vi "calc centroid predict and correct.vi"(0 "Queue in":refnum<queue>, 1 "Session Out":T2, 5 "# Images in Burst":i32, 11 "error in (no error)":errorcluster) -> (15 "error out":errorcluster)   [LabVIEW 2020]
uses:
  <vilib>/vision/Image Controls.llb/IMAQ Image.ctl
  <vilib>/userdefined/High Color/IMAQdx.ctl
  <vilib>/vision/driver/NI_Vision_Acquisition_Software.lvlib
panel:
  in  "Tab Control":enum32{"Page 1", "Page 2"}(tab)
  in  "Range":cluster{"Lower value":sgl, "Upper value":sgl}={"Lower value"=128.0, "Upper value"=255.0} caption="Threshold Range" {"Upper value" format="%.2f"; "Lower value" format="%.2f"}
  in  "Use threshold fraction":bool=TRUE
  out "Waveform Chart":T1(graph)
  out "Images Processed":u32
  out "# elements in queue":i32
  out "Current Buffer Number":u32
  out "processed in burst":u32
  in  "threshold fraction":sgl=0.8
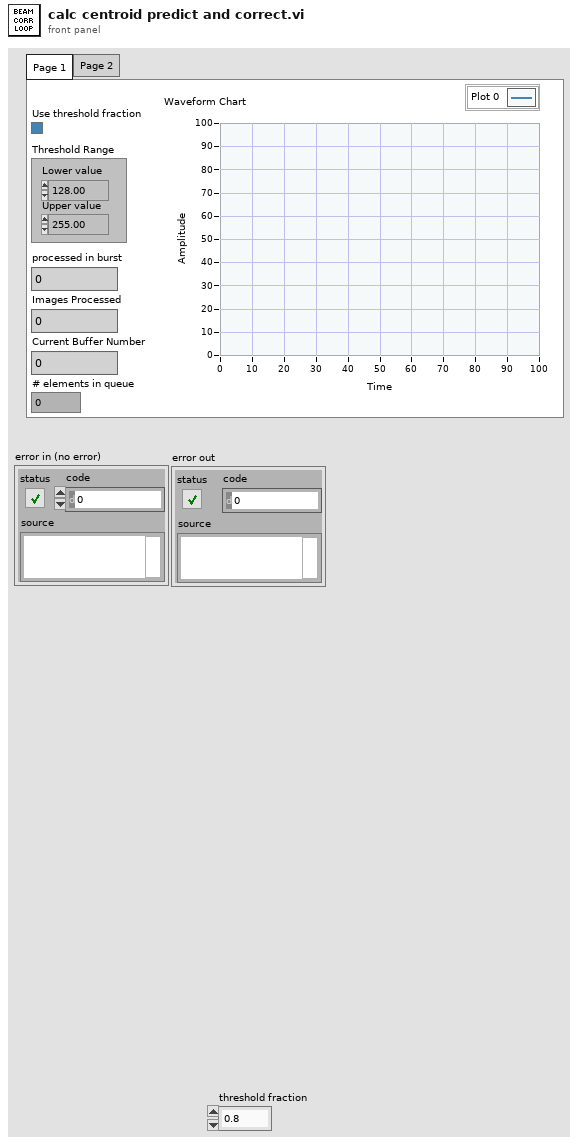
[diagram p1: front panel]
types:
  T1 = cluster{"X Centroid":sgl, "Y Centroid":sgl, "X Centroid":sgl, "Y Centroid":sgl}
  T2 = typedef "IMAQdx.ctl" = refnum<k21>
  T3 = typedef "IMAQ Image.ctl" = refnum<image>
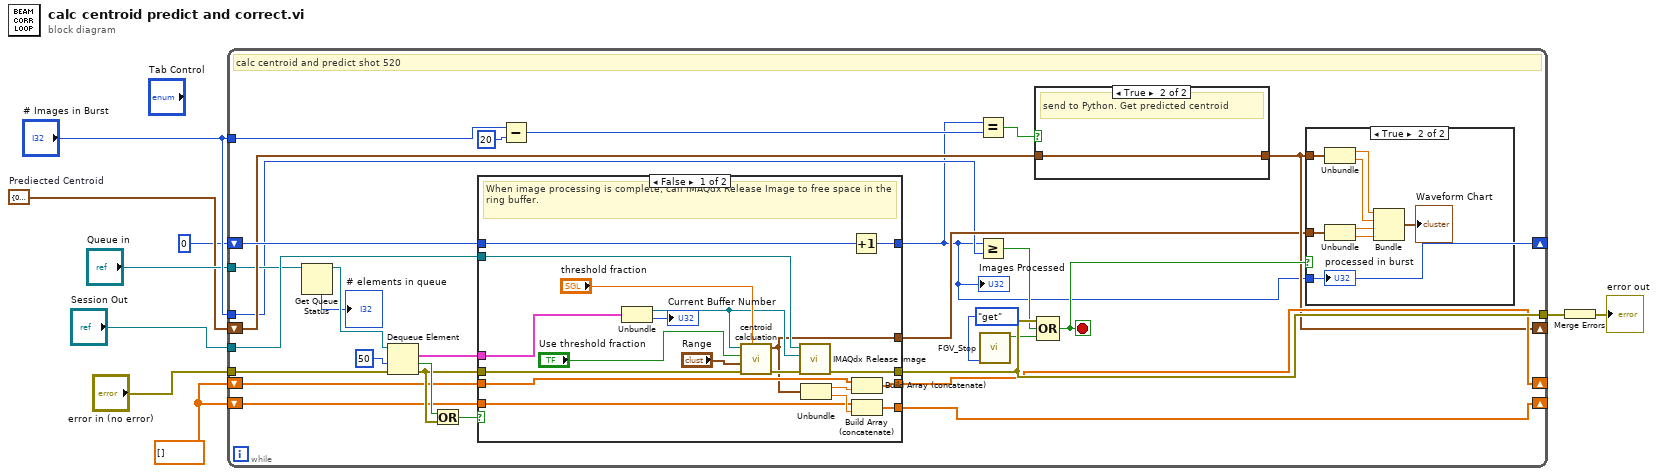
[diagram p0: block diagram]
diagram:
  w7 = cluster{"X Centroid":sgl, "Y Centroid":sgl} {"X Centroid"=0.0, "Y Centroid"=0.0}  # Prediected Centroid
  w6 = sgl[] []
  n1 = while {
    tunnel: [w29] -> w5
    tunnel: "Queue in" -> [w21]
    tunnel: "Session Out" -> [w36]
    shift-right: [w11] -> _
    shift-left: u32 0 -> [w35]
    tunnel: "error in (no error)" -> [w34]
    shift-right: [w27] -> _
    shift-left: w6 -> [w28]
    shift-right: [w26] -> _
    shift-left: w6 -> [w25]
    shift-right: [w23] -> _
    shift-left: w7 -> [w24]
    tunnel: "# Images in Burst" -> [w18]
    tunnel: "# Images in Burst" -> [w14]
    stop <- w30 stop-if-true
    # "calc centroid and predict shot 520"
    n2 = Get Queue Status(queue=w21) -> (queue out=w20:refnum<queue>, # elements in queue=→"# elements in queue":i32)  [unwired: 2 in, 6 out]
    n3 = Dequeue Element(queue=w20, timeout in ms (-1)=50 ("timeout in ms"), error in (no error)=w34) -> (element=w37:cluster{"Image Out":T3, "Buffer Number Out":u32}, timed out?=w32:bool, error out=w31:errorcluster)  [unwired: 1 out]
    n4 = Or(x=w32, y=w31) -> (x .or. y?=w33:bool)
    n5 = case shown="False" w33 {
      tunnel: w31 -> [w61 w71]
      tunnel: w37 -> [w67 _]
      tunnel: [w66 w71] -> w29
      tunnel: w36 -> [w65 _]
      tunnel: w35 -> [w63 w70]
      tunnel: [w62 w70] -> w11
      tunnel: w28 -> [w55 w69]
      tunnel: [w53 w69] -> w27
      tunnel: [w51 w68] -> w26
      tunnel: w25 -> [w50 w68]
      tunnel: [w49 _] -> w22
      frame False {
        # "When image processing is complete, call IMAQdx Release Image to free space in the ring buffer."
        n6 = Unbundle(w67) -> ("Image Out"=w58:T3, "Buffer Number Out"=→"Current Buffer Number":u32)
        n7 = call "centroid calcluation.vi"("threshold fraction"="threshold fraction", "error in (no error)"=w61, "Range"="Range", "Use threshold fraction"="Use threshold fraction", "Refnum in"=w58) -> ("error out"=w60:errorcluster, "Centroid"=w49:cluster{"X Centroid":sgl, "Y Centroid":sgl})  [unwired: 4 in, 1 out]
        n8 = call <vilib>:"IMAQdx Release Image.vi"("error in"=w60, "Image"=w58, "Session In"=w65) -> ("error out"=w66:errorcluster)  [unwired: 7 in, 1 out]
        n9 = Unbundle(w49) -> ("X Centroid"=w54:sgl, "Y Centroid"=w52:sgl)
        n10 = Increment(x=w63) -> (x+1=w62:u32)
        n11 = Build Array (concatenate)(w55, w54) -> (w53:sgl[])
        n12 = Build Array (concatenate)(w50, w52) -> (w51:sgl[])
      }
      frame True {
        # "Empty queue or error.\nNothing to process."
      }
    }
    "Images Processed" <- w11
    n13 = Subtract(x=w18, y=20) -> (x-y=w16:i32)
    n14 = Equal?(x=w11, y=w16) -> (x = y?=w10:bool)
    n15 = Greater Or Equal?(x=w11, y=w14) -> (x >= y?=w15:bool)
    n16 = call "FGV_Stop.vi"("command"=enum16{"set", "get"}."get") -> ("stop"=w12:bool)  [unwired: 10 in]
    n17 = case shown="True" w10 {
      tunnel: w24 -> [w39 w40]
      tunnel: [w39 w40] -> w23
      frame False {
      }
      frame True {
        # "send to Python. Get predicted centroid"
      }
    }
    n18 = Compound Arithmetic op=OR(w29, w15, w12) -> (w30:bool)
    n19 = case shown="True" w30 {
      tunnel: w23 -> [_ w47]
      tunnel: w22 -> [_ w48]
      tunnel: w11 -> [_ w41]
      frame False {
      }
      frame True {
        n20 = Unbundle(w47) -> ("X Centroid"=w46:sgl, "Y Centroid"=w45:sgl)
        n21 = Unbundle(w48) -> ("X Centroid"=w44:sgl, "Y Centroid"=w43:sgl)
        n22 = Bundle("X Centroid"=w46, "Y Centroid"=w45, "X Centroid"=w44, "Y Centroid"=w43) -> (→"Waveform Chart":T1)  [unwired: 1 in]
        "processed in burst" <- w41
      }
    }
  }
  n23 = Merge Errors(w5) -> (→"error out":errorcluster)
